vi "Teleop.vi"(10 "Match Info":T1={"Autonomous Elapsed Seconds"=0.0, "TeleOp Elapsed Seconds"=0.0, "Disabled Elapsed Seconds"=0.0, "Visited Autonomous"=FALSE, "Visited TeleOp"=FALSE, "Visited Disabled"=FALSE, "Autonomous Settings"={"Autonomous Style"=enum."Independent", "VI Refnum"=refnum}}, 11 "Call Context":T2) -> ()   [LabVIEW 2014]
doc: "This VI is called for each TeleOp packet received from the DS where the robot is not disabled. It is often used to read from the joysticks and update I/O or to update setpoints for timed control loops. It should complete and return within 20 milliseconds or it may miss DS packets."
uses:
  <vilib>/Rock Robotics/WPI/DriverStation/WPI_DriverStationDerivedRobotMode.ctl
  <vilib>/Rock Robotics/WPI/DriverStation/WPI_DriverStationMatch Info.ctl
  <vilib>/Rock Robotics/Network Tables/SD Read Boolean.vi
  <vilib>/Rock Robotics/Network Tables/SD Read Number.vi
  <vilib>/Rock Robotics/WPI/Joystick/WPI_JoystickGetSetRefNum.vi
  Robot Global Data.vi
  <vilib>/Rock Robotics/Network Tables/SD Write Number.vi
panel:
  out "Sample Slider 0":dbl(slide) scale=0.0..5.0
  out "Sample Boolean 1":bool
  out "Sample Boolean 0":bool
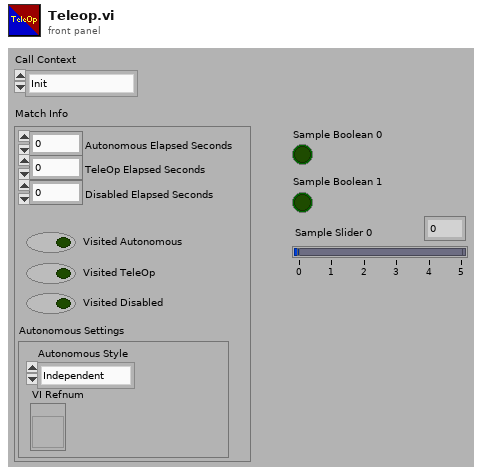
[diagram p1: front panel]
types:
  T1 = typedef "WPI_DriverStationMatch Info.ctl" = cluster{"Autonomous Elapsed Seconds":dbl, "TeleOp Elapsed Seconds":dbl, "Disabled Elapsed Seconds":dbl, "Visited Autonomous":bool, "Visited TeleOp":bool, "Visited Disabled":bool, "Autonomous Settings":cluster{"Autonomous Style":enum16{"Iterative", "Independent"}, "VI Refnum":refnum<vi>}}
  T2 = typedef "WPI_DriverStationDerivedRobotMode.ctl" = enum16{"Init", "Execute", "Stop"}
  T3 = typedef "WPI_JoystickDevRef.ctl" = cluster{"Device":T4}
  T4 = typedef "WPI_JoystickDeviceEnum.ctl" = enum16{"USB 0", "USB 1", "USB 2", "USB 3", "USB 4", "USB 5"}
  T5 = cluster{"Axes[0]":dbl, "Axes[1]":dbl, "Axes[2]":dbl, "Axes[3]":dbl, "Axes[4]":dbl, "Axes[5]":dbl, "Axes[6]":dbl, "Axes[7]":dbl, "Axes[8]":dbl}
  T6 = cluster{"Buttons[0]":bool, "Buttons[1]":bool, "Buttons[2]":bool, "Buttons[3]":bool, "Buttons[4]":bool, "Buttons[5]":bool, "Buttons[6]":bool, "Buttons[7]":bool, "Buttons[8]":bool}
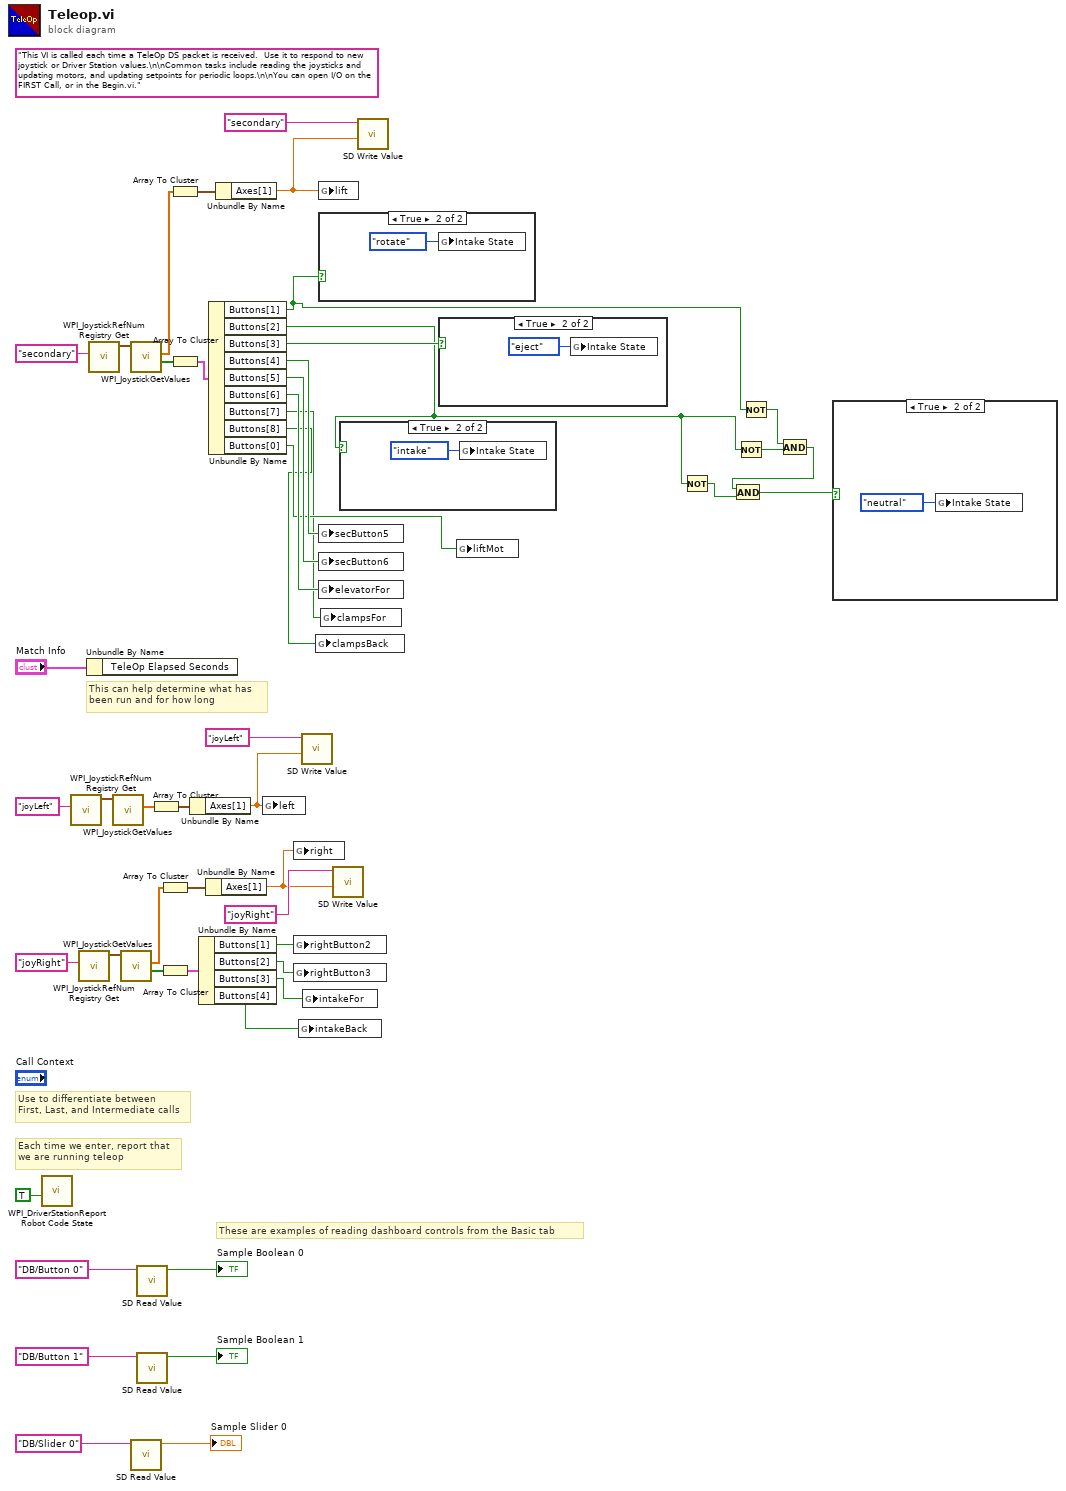
[diagram p0: block diagram]
diagram:
  (unwired) "This VI is called each time a TeleOp DS packet is received.  Use it to respond to new joystick or Driver Station values.\n\nCommon tasks include reading the joysticks and updating motors, and updating setpoints for periodic loops.\n\nYou can open I/O on the FIRST Call, or in the Begin.vi."
  # "These are examples of reading dashboard controls from the Basic tab"
  # "Each time we enter, report that\nwe are running teleop"
  # "Use to differentiate between\nFirst, Last, and Intermediate calls"
  # "This can help determine what has\nbeen run and for how long"
  n1 = call <vilib>:"WPI_DriverStationReport Robot Code State.vi"("TeleOp"=TRUE ("Autonomous")) -> ()  [unwired: 10 in, 1 out]
  n2 = call <vilib>:"WPI_JoystickRefNum Registry Get.vi"("refnum name"="joyLeft") -> ("JoystickDevRef"=w37:T3)  [unwired: 9 in, 1 out]
  n3 = call <vilib>:"WPI_JoystickRefNum Registry Get.vi"("refnum name"="joyRight") -> ("JoystickDevRef"=w40:T3)  [unwired: 9 in, 1 out]
  n4 = Unbundle By Name("Match Info") -> ()  [unwired: 1 out]
  n5 = call <vilib>:"WPI_JoystickRefNum Registry Get.vi"("refnum name"="secondary") -> ("JoystickDevRef"=w26:T3)  [unwired: 9 in, 1 out]
  n6 = call <vilib>:"WPI_JoystickGetValues.vi"("JoystickDevRef"=w37) -> ("Axes"=w36:dbl[])  [unwired: 6 in, 4 out]
  n7 = call <vilib>:"WPI_JoystickGetValues.vi"("JoystickDevRef"=w40) -> ("Buttons"=w31:bool[], "Axes"=w34:dbl[])  [unwired: 6 in, 3 out]
  n8 = call <vilib>:"WPI_JoystickGetValues.vi"("JoystickDevRef"=w26) -> ("Buttons"=w24:bool[], "Axes"=w27:dbl[])  [unwired: 6 in, 3 out]
  n9 = call-poly <vilib>:"SD Read Value.vi"("Name"="DB/Slider 0" ("refnum name")) -> ("Numeric"=→"Sample Slider 0":dbl)  [unwired: 8 in, 2 out]
  n10 = call-poly <vilib>:"SD Read Value.vi"("Name"="DB/Button 0" ("refnum name")) -> ("Boolean"=→"Sample Boolean 0":bool)  [unwired: 8 in, 2 out]
  n11 = call-poly <vilib>:"SD Read Value.vi"("Name"="DB/Button 1" ("refnum name")) -> ("Boolean"=→"Sample Boolean 1":bool)  [unwired: 8 in, 2 out]
  n12 = Array To Cluster(array=w36) -> (cluster=w35:T5)
  n13 = Array To Cluster(array=w34) -> (cluster=w33:T5)
  n14 = Array To Cluster(array=w31) -> (cluster=w32:T6)
  n15 = Array To Cluster(array=w27) -> (cluster=w28:T5)
  n16 = Array To Cluster(array=w24) -> (cluster=w23:T6)
  n17 = Unbundle By Name(w35) -> ("Axes[1]"=w19:dbl)
  n18 = Unbundle By Name(w32) -> ("Buttons[1]"=w30:bool, "Buttons[2]"=w29:bool, "Buttons[3]"=w2:bool, "Buttons[4]"=w1:bool)
  n19 = Unbundle By Name(w33) -> ("Axes[1]"=w16:dbl)
  n20 = Unbundle By Name(w23) -> ("Buttons[1]"=w11:bool, "Buttons[2]"=w10:bool, "Buttons[3]"=w12:bool, "Buttons[4]"=w22:bool, "Buttons[5]"=w21:bool, "Buttons[6]"=w20:bool, "Buttons[7]"=w4:bool, "Buttons[8]"=w3:bool, "Buttons[0]"=w13:bool)
  n21 = Unbundle By Name(w28) -> ("Axes[1]"=w14:dbl)
  n22 = global write "Robot Global Data.vi" "left"(w19) -> ()
  n23 = global write "Robot Global Data.vi" "right"(w16) -> ()
  n24 = global write "Robot Global Data.vi" "rightButton2"(w30) -> ()
  n25 = global write "Robot Global Data.vi" "rightButton3"(w29) -> ()
  n26 = global write "Robot Global Data.vi" "intakeBack"(w1) -> ()
  n27 = call-poly <vilib>:"SD Write Value.vi"("Numeric"=w19, "Name"="joyLeft") -> ()  [unwired: 8 in, 2 out]
  n28 = global write "Robot Global Data.vi" "intakeFor"(w2) -> ()
  n29 = global write "Robot Global Data.vi" "clampsBack"(w3) -> ()
  n30 = global write "Robot Global Data.vi" "lift"(w14) -> ()
  n31 = case shown="True" w11 {
    frame False {
    }
    frame True {
      n32 = global write "Robot Global Data.vi" "Intake State"(enum16{"neutral", "rotate", "intake", "eject"}."rotate" ("Intake State")) -> ()
    }
  }
  n33 = global write "Robot Global Data.vi" "secButton5"(w22) -> ()
  n34 = global write "Robot Global Data.vi" "secButton6"(w21) -> ()
  n35 = global write "Robot Global Data.vi" "elevatorFor"(w20) -> ()
  n36 = global write "Robot Global Data.vi" "clampsFor"(w4) -> ()
  n37 = call-poly <vilib>:"SD Write Value.vi"("Numeric"=w16, "Name"="joyRight") -> ()  [unwired: 8 in, 2 out]
  n38 = case shown="True" w10 {
    frame False {
    }
    frame True {
      n39 = global write "Robot Global Data.vi" "Intake State"(enum16{"neutral", "rotate", "intake", "eject"}."intake" ("Intake State")) -> ()
    }
  }
  n40 = call-poly <vilib>:"SD Write Value.vi"("Numeric"=w14, "Name"="secondary") -> ()  [unwired: 8 in, 2 out]
  n41 = case shown="True" w12 {
    frame False {
    }
    frame True {
      n42 = global write "Robot Global Data.vi" "Intake State"(enum16{"neutral", "rotate", "intake", "eject"}."eject" ("Intake State")) -> ()
    }
  }
  n43 = global write "Robot Global Data.vi" "liftMot"(w13) -> ()
  n44 = Not(x=w10) -> (.not. x?=w7:bool)
  n45 = Not(x=w10) -> (.not. x?=w8:bool)
  n46 = Not(x=w11) -> (.not. x?=w9:bool)
  n47 = And(x=w9, y=w8) -> (x .and. y?=w6:bool)
  n48 = And(x=w6, y=w7) -> (x .and. y?=w5:bool)
  n49 = case shown="True" w5 {
    frame False {
    }
    frame True {
      n50 = global write "Robot Global Data.vi" "Intake State"(enum16{"neutral", "rotate", "intake", "eject"}."neutral" ("Intake State")) -> ()
    }
  }
